vi "Time_Global.vi"(8 "Time Stamp In":timestamp, 9 "Time Stamp Select":T1, 11 "ID":i32=-1) -> (1 "Time (S)":dbl, 3 "ID Out":i32)   [LabVIEW 2020]
uses:
  TypeDefs/ENUM_Time Type Select.ctl
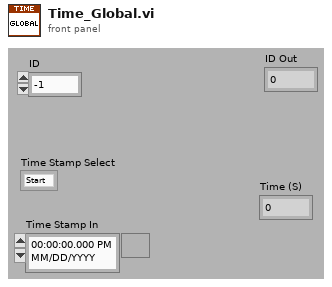
[diagram p1: front panel]
types:
  T1 = typedef "ENUM_Time Type Select.ctl" = enum16{"Start", "Time", "Cycle"}
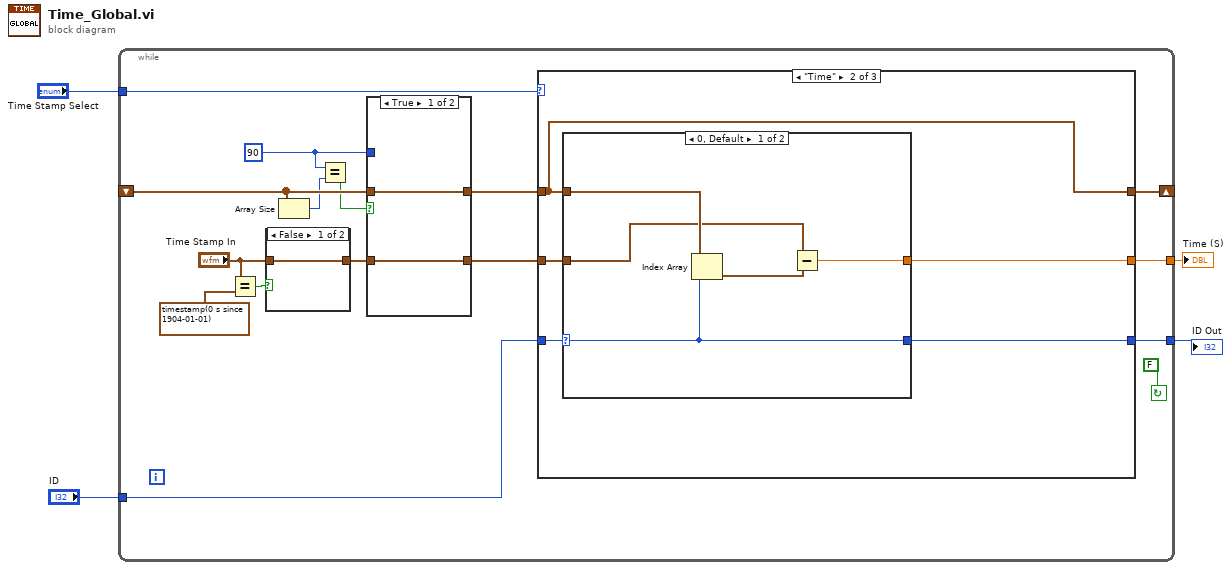
[diagram p0: block diagram]
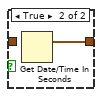
[diagram p2: hidden frame]
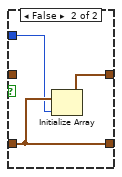
[diagram p3: hidden frame]
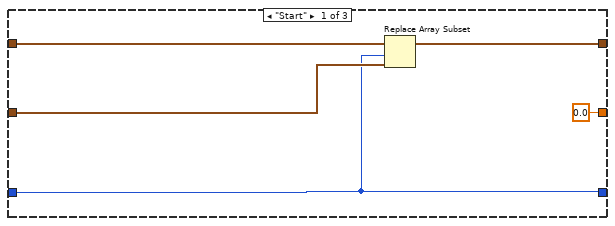
[diagram p4: hidden frame]
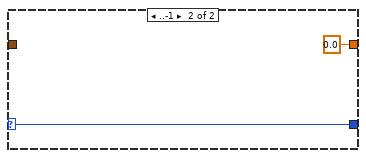
[diagram p5: hidden frame]
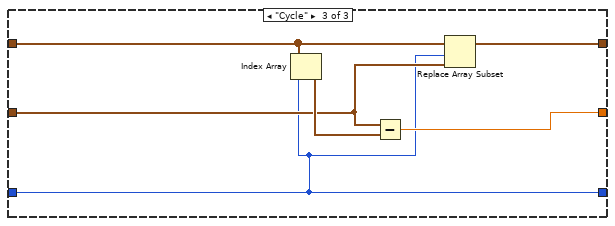
[diagram p6: hidden frame]
diagram:
  n1 = while {
    shift-right: [w19] -> _
    shift-left: _ -> [w15]
    tunnel: "Time Stamp Select" -> [w20]
    tunnel: [w18] -> w3
    tunnel: "ID" -> [w12]
    tunnel: [w11] -> w1
    stop <- FALSE continue-if-true
    w6 = 90 ("dimension size")
    n2 = Equal?(x="Time Stamp In", y=timestamp(0 s since 1904-01-01) ("Time Stamp")) -> (x = y?=w10:bool)
    n3 = case shown="False" w10 {
      tunnel: [w21 w22] -> w14
      tunnel: "Time Stamp In" -> [w21 _]
      frame False {
      }
      frame True {
        n4 = Get Date/Time In Seconds() -> (seconds since 1Jan1904=w22:timestamp)
      }
    }
    n5 = Array Size(array=w15) -> (size(s)=w7:i32)
    n6 = Equal?(x=w6, y=w7) -> (x = y?=w5:bool)
    n7 = case shown="True" w5 {
      tunnel: w15 -> [w24 _]
      tunnel: [w24 w27] -> w16
      tunnel: w14 -> [w23 w26]
      tunnel: [w23 w26] -> w13
      tunnel: w6 -> [_ w25]
      frame True {
      }
      frame False {
        n8 = Initialize Array(w26, w25) -> (w27:timestamp[])
      }
    }
    n9 = case shown="\"Time\"" w20 {
      tunnel: [w30 w36 w47] -> w19
      tunnel: w16 -> [w31 w36 w48]
      tunnel: [0.0 w33 w49] -> w18
      tunnel: w12 -> [w28 w35 w45]
      tunnel: w13 -> [w29 w37 w46]
      tunnel: [w28 w34 w45] -> w11
      frame "Start" {
        n10 = Replace Array Subset(array=w31, new element=w29, index=w28) -> (w30:timestamp[])
      }
      frame "Time" {
        n11 = case shown="0, Default" w35 {
          selector: w35 -> [w38 w43]
          tunnel: [w41 0.0] -> w33
          tunnel: w36 -> [w40 _]
          tunnel: w37 -> [w39 _]
          tunnel: [w38 w43] -> w34
          frame 0, Default {
            n12 = Index Array(array=w40, index=w38) -> (element=w42:timestamp)
            n13 = Subtract(x=w39, y=w42) -> (x-y=w41:dbl)
          }
          frame ..-1 {
          }
        }
      }
      frame "Cycle" {
        n14 = Index Array(array=w48, index=w45) -> (element=w50:timestamp)
        n15 = Subtract(x=w46, y=w50) -> (x-y=w49:dbl)
        n16 = Replace Array Subset(array=w48, new element=w46, index=w45) -> (w47:timestamp[])
      }
    }
  }
  "Time (S)" <- w3
  "ID Out" <- w1
